vi "FGVOscilloscope.vi"(7 "Enum":T1, 8 "error in":errorcluster, 9 "NextChannelIn":i32, 10 "LastValuesIn":dbl[](array[numeric])) -> (0 "error out":errorcluster, 1 "NextChannelOut":i32, 2 "LastValuesOut":dbl[](array[numeric]))   [LabVIEW 2016]
uses:
  controls/Enum.ctl
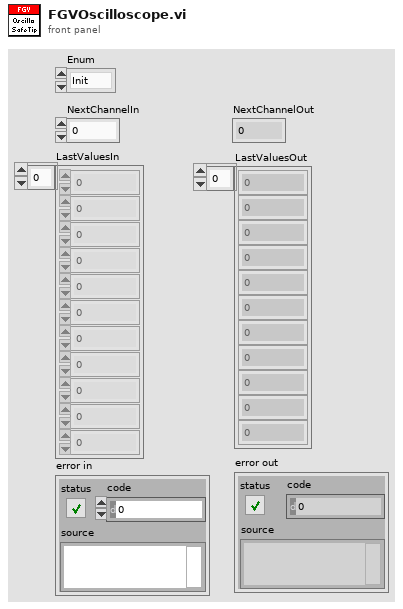
[diagram p1: front panel]
types:
  T1 = typedef "Enum.ctl" = enum16{"Init", "Read", "Write"}
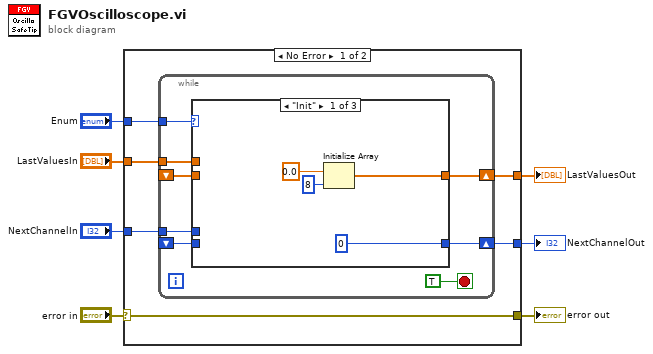
[diagram p0: block diagram]
diagram:
  n1 = case shown="No Error" "error in" {
    selector: "error in" -> [w12 w32]
    tunnel: "Enum" -> [w13 _]
    tunnel: [w12 w32] -> w6
    tunnel: "NextChannelIn" -> [w11 w31]
    tunnel: [w10 w31] -> w1
    tunnel: [w9 w30] -> w4
    tunnel: "LastValuesIn" -> [w8 w30]
    frame No Error {
      n2 = while {
        tunnel: w13 -> [w20]
        tunnel: w11 -> [w19]
        shift-right: [w18] -> w10
        shift-left: _ -> [w17]
        shift-right: [w16] -> w9
        shift-left: _ -> [w14]
        tunnel: w8 -> [w15]
        stop <- TRUE stop-if-true
        n3 = case shown="\"Init\"" w20 {
          tunnel: w19 -> [_ _ w28]
          tunnel: [0 w27 w28] -> w18
          tunnel: w17 -> [_ w27 _]
          tunnel: [w23 w26 w29] -> w16
          tunnel: w15 -> [_ _ w29]
          tunnel: w14 -> [_ w26 _]
          frame "Init" {
            n4 = Initialize Array(0.0 ("element"), 8 ("dimension size")) -> (w23:dbl[])
          }
          frame "Read", Default {
          }
          frame "Write" {
          }
        }
      }
    }
    frame Error {
    }
  }
  "error out" <- w6
  "LastValuesOut" <- w4
  "NextChannelOut" <- w1
